vi "controlMotionControlThreshold.vi"(7 "Set":bool, 8 "error in":errorcluster, 9 "threshold [nm]":i32, 10 "axis in":u8, 11 "connection ID":refnum<k5>) -> (0 "error out":errorcluster, 1 "threshold out":i32, 2 "axis out":u8, 3 "connection ID":refnum<k5>)   [LabVIEW 2015, in "AMC_VIs.lvlib"]
doc: "This function retrieves or sets the threshold range within the closed-loop controlled movement stops to regulate."
uses:
  AMC_VIs.lvlib
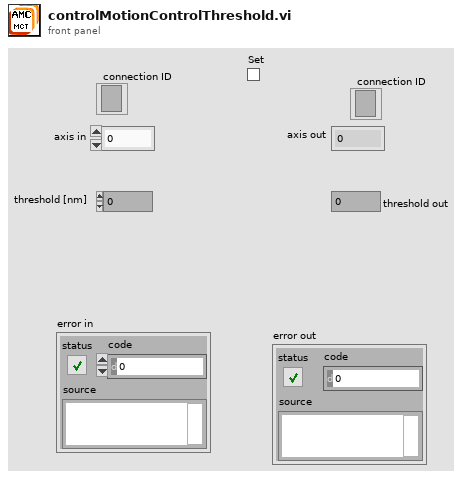
[diagram p1: front panel]
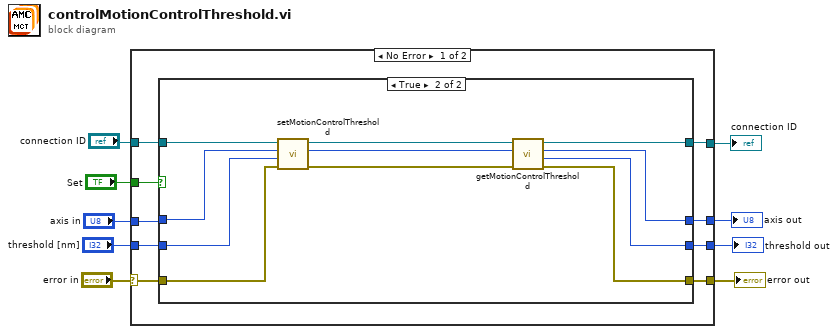
[diagram p0: block diagram]
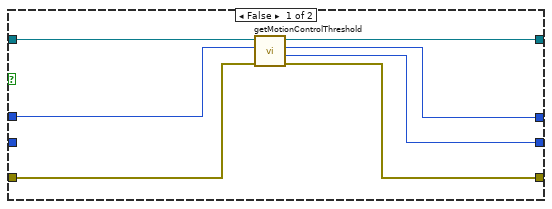
[diagram p2: hidden frame]
diagram:
  n1 = case shown="No Error" "error in" {
    selector: "error in" -> [w12 w40]
    tunnel: "axis in" -> [w16 w39]
    tunnel: [w13 w40] -> w8
    tunnel: [w14 w39] -> w7
    tunnel: "Set" -> [w17 _]
    tunnel: [w15 w38] -> w5
    tunnel: "connection ID" -> [w18 w38]
    tunnel: "threshold [nm]" -> [w11 w37]
    tunnel: [w10 w37] -> w1
    frame No Error {
      n2 = case shown="True" w17 {
        tunnel: [w24 w26] -> w15
        tunnel: w18 -> [w25 w36]
        tunnel: w16 -> [w23 w34]
        tunnel: [w22 w27] -> w14
        tunnel: [w20 w29] -> w13
        tunnel: w12 -> [w21 w35]
        tunnel: w11 -> [_ w33]
        tunnel: [w19 w28] -> w10
        frame False {
          n3 = call "getMotionControlThreshold.vi"("error in"=w21, "axis"=w23, "connection ID"=w25) -> ("error out"=w20:errorcluster, "range"=w19:i32, "axis_out"=w22:i32, "connection ID"=w24:refnum<k5>)  [unwired: 5 in]
        }
        frame True {
          n4 = call "setMotionControlThreshold.vi"("error in"=w35, "threshold"=w33, "axis"=w34, "connection ID"=w36) -> ("error out"=w30:errorcluster, "axis_out"=w31:i32, "connection ID"=w32:refnum<k5>)  [unwired: 5 in]
          n5 = call "getMotionControlThreshold.vi"("error in"=w30, "axis"=w31, "connection ID"=w32) -> ("error out"=w29:errorcluster, "range"=w28:i32, "axis_out"=w27:i32, "connection ID"=w26:refnum<k5>)  [unwired: 5 in]
        }
      }
    }
    frame Error {
    }
  }
  "error out" <- w8
  "axis out" <- w7
  "connection ID" <- w5
  "threshold out" <- w1
